vi "Read Text labels visible.vi"(9 "NumericWithScale in":refnum<class "NumericWithScale.lvclass">) -> (3 "NumericWithScale out":refnum<class "NumericWithScale.lvclass">, 4 "Text labels visible":bool)   [LabVIEW 2014, in "NumericWithScale.lvclass"]
uses:
  NumericWithScale.lvclass
  NumericWithScale.lvclass/NumericWithScale.ctl
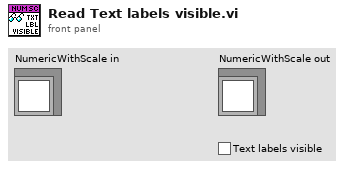
[diagram p1: front panel]
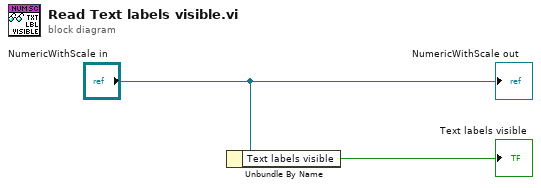
[diagram p0: block diagram]
diagram:
  n1 = Unbundle By Name("NumericWithScale in") -> ("Text labels visible"=→"Text labels visible":bool)
  "NumericWithScale out" <- "NumericWithScale in"
